vi "PanelClose.vi"(8 "error in (no error)":errorcluster, 11 "DAQ_Module in":refnum<class "DAQ_Module.lvclass">) -> (0 "error out":errorcluster, 3 "DAQ_Module out":refnum<class "DAQ_Module.lvclass">)   [LabVIEW 2025, in "DAQ_Module.lvlib" / "DAQ_Module.lvclass"]
uses:
  DAQ_Module.lvclass
  Msg.ctl
  DAQ_Module.lvclass/DAQ_Module.ctl
  Read Debug.vi
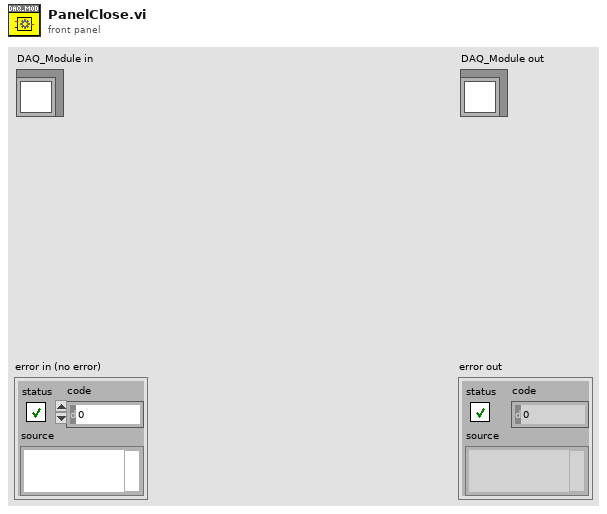
[diagram p1: front panel]
types:
  T1 = typedef "Msg.ctl" = string
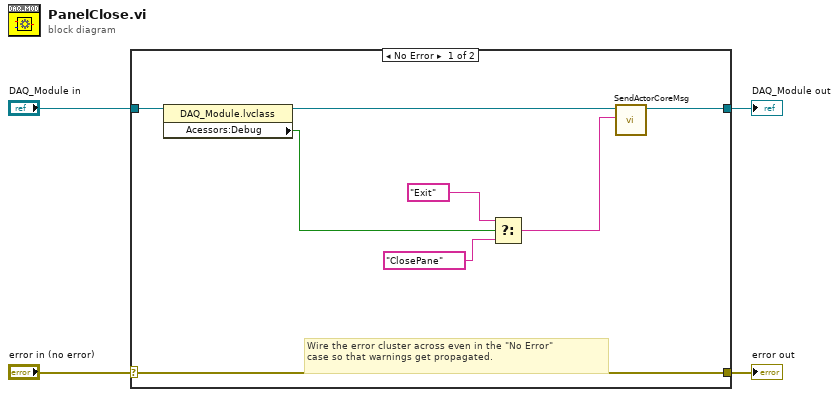
[diagram p0: block diagram]
diagram:
  n1 = case shown="No Error" "error in (no error)" {
    selector: "error in (no error)" -> [w11 w14]
    tunnel: [w11 w14] -> w3
    tunnel: [w6 w13] -> w1
    tunnel: "DAQ_Module in" -> [w12 w13]
    frame No Error {
      # "Wire the error cluster across even in the \"No Error\"\ncase so that warnings get propagated."
      n2 = property class="DAQ_Module.lvclass"(reference=w12) -> (reference out=w7:refnum<class "DAQ_Module.lvclass">, "Acessors:Debug"=w8:bool)  [unwired: 1 in, 1 out]
      n3 = Select(t=T1 "Exit" ("Msg"), s=w8, f=T1 "ClosePane" ("Msg")) -> (s? t:f=w5:T1)
      n4 = call "SendActorCoreMsg.vi"("Msg"=w5, "DAQ_Module in"=w7) -> ("DAQ_Module out"=w6:refnum<class "DAQ_Module.lvclass">)  [unwired: 8 in, 1 out]
    }
    frame Error {
    }
  }
  "error out" <- w3
  "DAQ_Module out" <- w1
